vi "Ballard 429 - Build Message.vi"(0 "Channel Data []":T5[](array[typedef])=[{"Labels Settings"=[{"Name"="", "xmlName"="", "Label"=0, "transferPeriod"=0, "SDI_Enabled"=FALSE, "SDI"=0, "Word"={"Param Setting"={"Start Bit"=[], "Num Bits"=[], "Signed?"=[], "ScaleFac"=[], "ScaleOffset"=[], "Block Data Refs"=[], "Encoding"=[], "Values Array"=[], "Item Refs"=[]}}, "TransferType"=enum."ScheduledLabel", "has timestamp?"=FALSE, "Label Disable/Trigger Channel Reference"=0, "Message Handle"=0, "Initialized?"=FALSE, "Word Initial Raw Value"=0, "Label Timestamp Channel Data Reference"=0}], "channel handle"=0, "channel #"=0}] {"Labels Settings"."Label Timestamp Channel Data Reference" format="%.0x"; "Labels Settings"."Label Disable/Trigger Channel Reference" format="%.0x"; "Labels Settings"."Word"."Param Setting"."Item Refs" format="%.0x"; "Labels Settings"."Word"."Param Setting"."Num Bits" min=1 max=32; "Labels Settings"."Word"."Param Setting"."Start Bit" min=8 max=31; "Labels Settings"."Label" format="%.0o"}, 5 "Doubles []":dbl[](array[numeric]), 9 "Updated FIFO Index []":i32[](array[numeric]), 11 "Error (in)":errorcluster, 12 "Map":T4[](array[typedef]) {"Channel Data Reference" format="%.0x"}, 13 "Raw Values":T1) -> (15 "Error (out)":errorcluster)   [LabVIEW 2019, in "Ballard Arinc-429 Engine.lvlib"]
uses:
  Ballard Arinc-429 Engine.lvlib
  Shared/Controls and Global/RT HW Channel.ctl
  Shared/Controls and Global/RT Label Settings.ctl
  Shared/Controls and Global/Label.ctl
  Shared/Controls and Global/transferPeriod.ctl
  Shared/Controls and Global/RT Word Settings.ctl
  Shared/Controls and Global/RT Param Setting.ctl
  Shared/Controls and Global/Start Bit.ctl
  Shared/Controls and Global/Number of Bits.ctl
  <vilib>/NI VeriStand/Custom Device API/Block Data Reference.ctl
  <vilib>/NI VeriStand/Custom Device API/Data Reference.ctl
  <vilib>/NI VeriStand/Custom Device API/Custom Device Item Ref.ctl
  Shared/Controls and Global/TransferType.ctl
  RT Controls/RT Tx Association.ctl
  RT Controls/RT Tx Default Raw Value.ctl
  RT Controls/RT Tx Default Raw Value_Association.ctl
  Insert BCD Parameter.vi
  <instrlib>/BTI429Lib/BTI429LV.lvlib
  <vilib>/NI VeriStand/Custom Device Tools/Custom Device Utility Library/Custom Device Utility Library.lvlib
  Shared/Ballard Arinc-429 Shared.lvlib
  <vilib>/NI VeriStand/Custom Device API/Custom Device API.lvlib
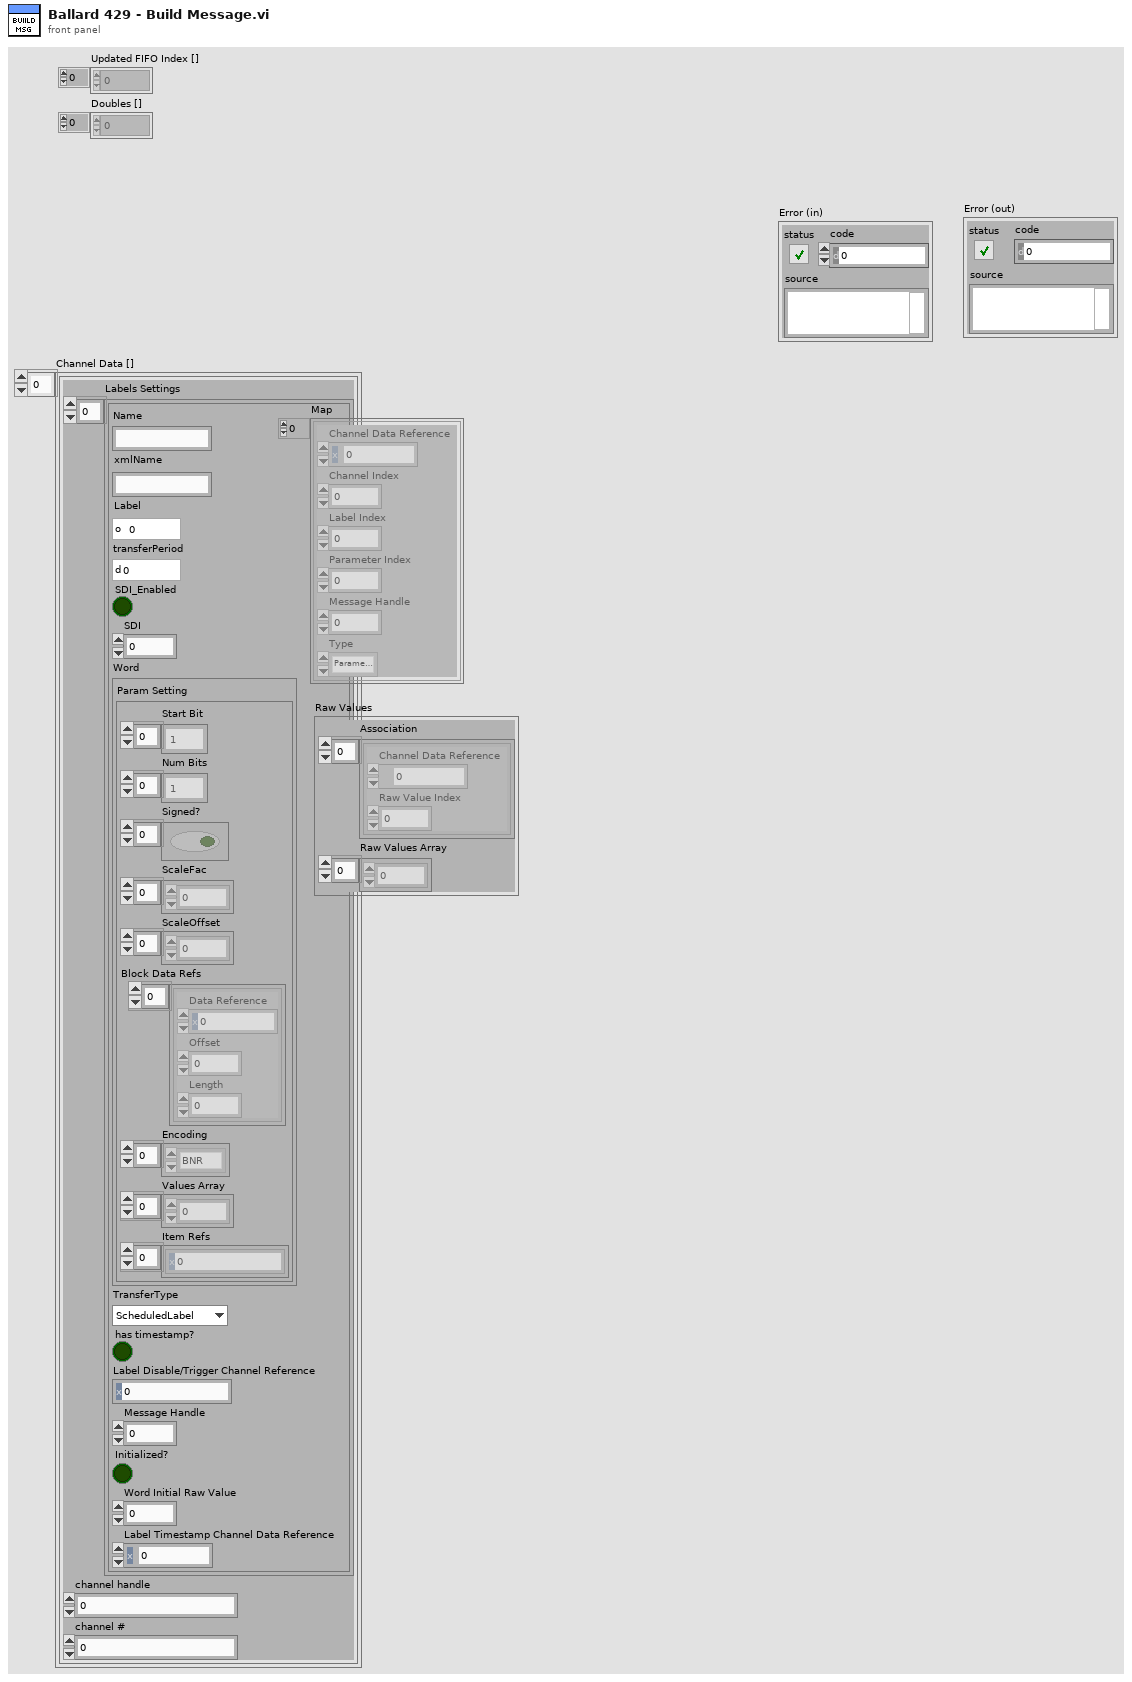
[diagram p1: front panel]
types:
  T1 = typedef "Ballard Arinc-429 Engine.lvlib/RT Tx Default Raw Value.ctl" = cluster{"Association":T2[], "Raw Values Array":u32[]}
  T2 = typedef "Ballard Arinc-429 Engine.lvlib/RT Tx Default Raw Value_Association.ctl" = cluster{"Channel Data Reference":T3, "Raw Value Index":i32}
  T3 = typedef "Custom Device API.lvlib/Data Reference.ctl" = i32
  T4 = typedef "Ballard Arinc-429 Engine.lvlib/RT Tx Association.ctl" = cluster{"Channel Data Reference":T3, "Channel Index":i32, "Label Index":i32, "Parameter Index":i32, "Message Handle":u64, "Type":enum16{"Parameter Channel", "Disable/Trigger Channel"}}
  T5 = typedef "Ballard Arinc-429 Shared.lvlib/RT HW Channel.ctl" = cluster{"Labels Settings":T6[], "channel handle":u64, "channel #":u16}
  T6 = typedef "Ballard Arinc-429 Shared.lvlib/RT Label Settings.ctl" = cluster{"Name":string, "xmlName":string, "Label":T7, "transferPeriod":T8, "SDI_Enabled":bool, "SDI":u8, "Word":T9, "TransferType":T15, "has timestamp?":bool, "Label Disable/Trigger Channel Reference":T14, "Message Handle":u64, "Initialized?":bool, "Word Initial Raw Value":u32, "Label Timestamp Channel Data Reference":T3}
  T7 = typedef "Ballard Arinc-429 Shared.lvlib/Label.ctl" = u8
  T8 = typedef "Ballard Arinc-429 Shared.lvlib/transferPeriod.ctl" = u32
  T9 = typedef "Ballard Arinc-429 Shared.lvlib/RT Word Settings.ctl" = cluster{"Param Setting":T10}
  T10 = typedef "Ballard Arinc-429 Shared.lvlib/RT Param Setting.ctl" = cluster{"Start Bit":T11[], "Num Bits":T12[], "Signed?":bool[], "ScaleFac":dbl[], "ScaleOffset":dbl[], "Block Data Refs":T13[], "Encoding":enum16{"BNR", "BCD", "Discrete"}[], "Values Array":dbl[], "Item Refs":T14[]}
  T11 = typedef "Ballard Arinc-429 Shared.lvlib/Start Bit.ctl" = i32
  T12 = typedef "Ballard Arinc-429 Shared.lvlib/Number of Bits.ctl" = i32
  T13 = typedef "Custom Device API.lvlib/Block Data Reference.ctl" = cluster{"Data Reference":T3, "Offset":u64, "Length":u64}
  T14 = typedef "Custom Device API.lvlib/Custom Device Item Ref.ctl" = u64
  T15 = typedef "Ballard Arinc-429 Shared.lvlib/TransferType.ctl" = enum16{"ScheduledLabel", "Acyclic", "Block", "Strobe"}
  T16 = enum16{"Parameter Channel", "Disable/Trigger Channel"}
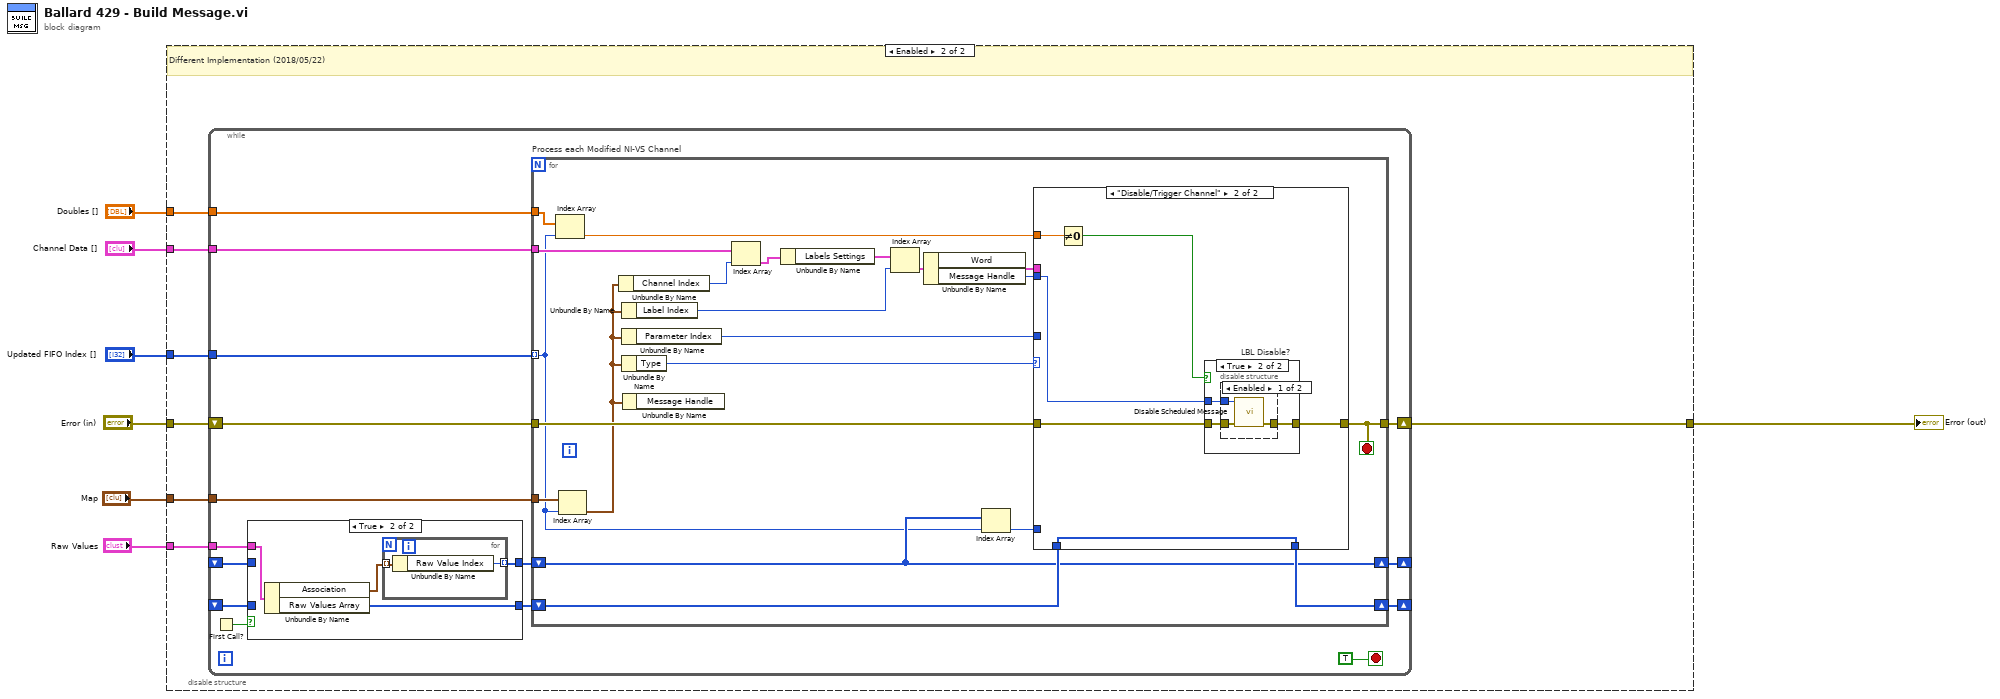
[diagram p0: block diagram]
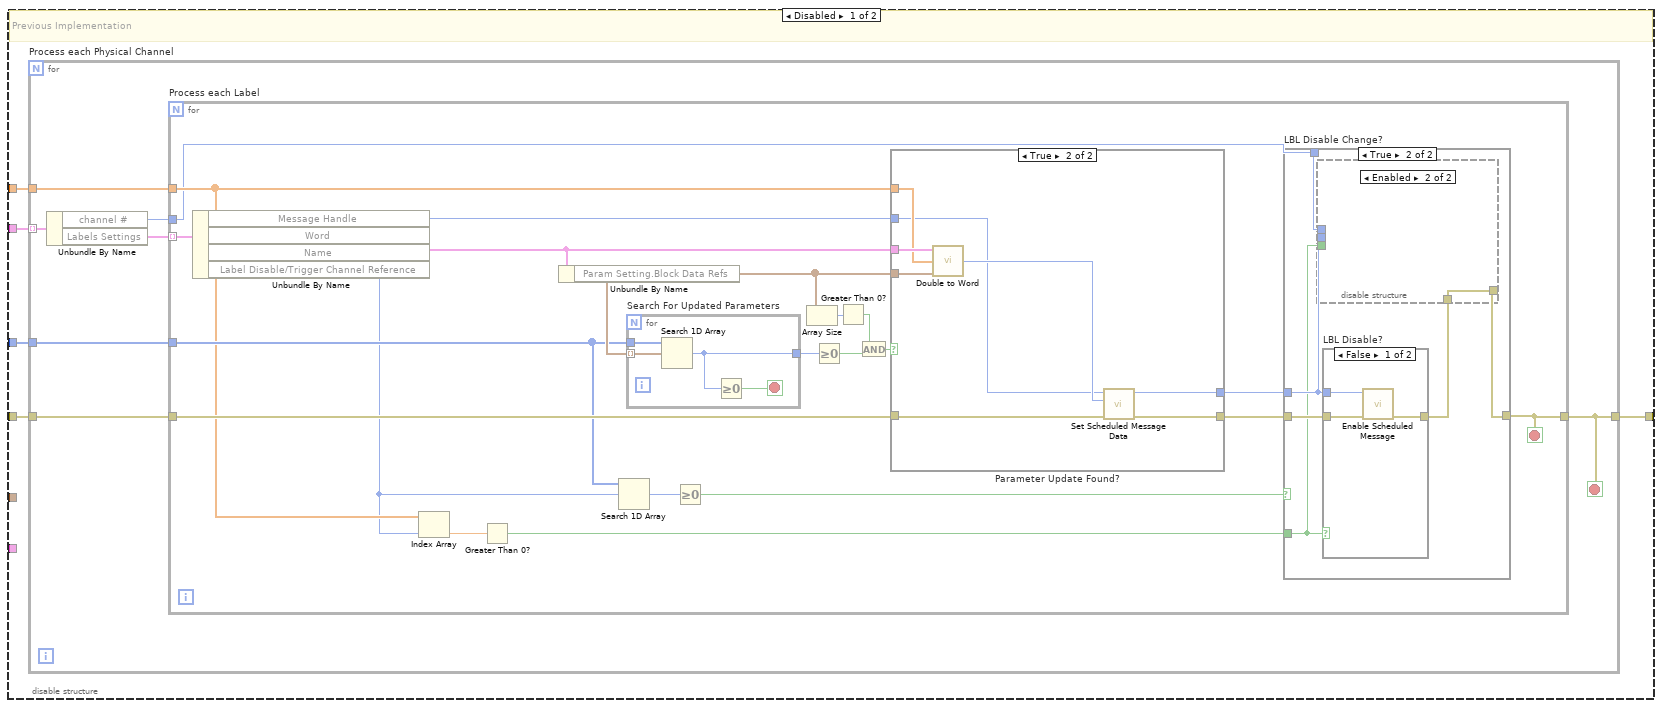
[diagram p2: hidden frame]
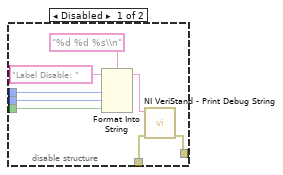
[diagram p4: hidden frame]
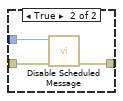
[diagram p5: hidden frame]
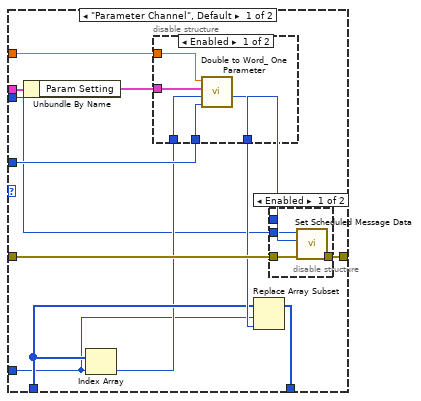
[diagram p8: hidden frame]
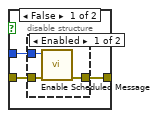
[diagram p11: hidden frame]
diagram:
  n1 = disable-structure shown="Enabled" {
    disable-tunnel: "Channel Data []" -> [w12 w83]
    disable-tunnel: "Updated FIFO Index []" -> [w11 w82]
    disable-tunnel: "Error (in)" -> [w10 w81]
    disable-tunnel: [w9 w80] -> w4
    disable-tunnel: "Doubles []" -> [w8 w79]
    disable-tunnel: "Map" -> [_ w78]
    disable-tunnel: "Raw Values" -> [_ w77]
    frame Disabled {
      # "Previous Implementation"
      n2 = for "Process each Physical Channel" {
        tunnel: w12 -> [w19] mode=indexing
        tunnel: w11 -> [w17]
        tunnel: w8 -> [w16]
        tunnel: w10 -> [w15]
        tunnel: [w14] -> w9
        stop <- w14 stop-if-true
        n3 = Unbundle By Name(w19) -> ("channel #"=w13:u16, "Labels Settings"=w18:T6[])
        n4 = for "Process each Label" {
          tunnel: w18 -> [w40] mode=indexing
          tunnel: w17 -> [w32]
          tunnel: w16 -> [w27]
          tunnel: [w29] -> w14
          tunnel: w15 -> [w38]
          tunnel: w13 -> [w21]
          stop <- w29 stop-if-true
          n5 = Unbundle By Name(w40) -> ("Message Handle"=w22:u64, "Word"=w20:T9, "Label Disable/Trigger Channel Reference"=w26:T14)  [unwired: 1 out]
          n6 = Index Array(array=w27, index=w26) -> (element=w25:dbl)
          n7 = Greater Than 0?(x=w25) -> (x > 0?=w24:bool)
          n8 = Unbundle By Name(w20) -> ("Param Setting.Block Data Refs"=w37:T13[])
          n9 = Search 1D Array(1D array=w32, element=w26) -> (index of element=w31:i32)  [unwired: 1 in]
          n10 = for "Search For Updated Parameters" {
            tunnel: w32 -> [w76]
            tunnel: w37 -> [w75] mode=indexing
            tunnel: [w74] -> w39
            stop <- w73 stop-if-true
            n11 = Search 1D Array(1D array=w76, element=w75) -> (index of element=w74:i32)  [unwired: 1 in]
            n12 = Greater Or Equal To 0?(x=w74) -> (x >= 0?=w73:bool)
          }
          n13 = Greater Or Equal To 0?(x=w31) -> (x >= 0?=w30:bool)
          n14 = Array Size(array=w37) -> (size(s)=w36:i32)
          n15 = Greater Or Equal To 0?(x=w39) -> (x >= 0?=w34:bool)
          n16 = Greater Than 0?(x=w36) -> (x > 0?=w35:bool)
          n17 = And(x=w35, y=w34) -> (x .and. y?=w33:bool)
          n18 = case "Parameter Update Found?" shown="True" w33 {
            tunnel: w27 -> [_ w68]
            tunnel: w20 -> [_ w72]
            tunnel: w38 -> [w64 w67]
            tunnel: [w64 w71] -> w28
            tunnel: w37 -> [_ w69]
            tunnel: w22 -> [w63 w66]
            tunnel: [w63 w65] -> w23
            frame False {
            }
            frame True {
              n19 = call "Double to Word.vi"("Word"=w72, "Doubles In []"=w68, "Channel FIFO Buffer Index"=w69) -> ("Word"=w70:u32)  [unwired: 12 in]
              n20 = call <instrlib>:"Set Scheduled Message Data.vi"("error in (no error)"=w67, "value"=w70, "message handle in"=w66) -> ("error out"=w71:errorcluster, "message handle out"=w65:u64)  [unwired: 7 in]
            }
          }
          n21 = case "LBL Disable Change?" shown="True" w30 {
            tunnel: [w41 w46] -> w29
            tunnel: w28 -> [w41 w47]
            tunnel: w24 -> [_ w42]
            tunnel: w23 -> [_ w43]
            tunnel: w21 -> [_ w44]
            frame False {
            }
            frame True {
              n22 = case "LBL Disable?" shown="False" w42 {
                tunnel: [w59 w62] -> w45
                tunnel: w47 -> [w58 w61]
                tunnel: w43 -> [w57 w60]
                frame False {
                  n23 = call <instrlib>:"Enable Scheduled Message.vi"("error in (no error)"=w58, "message handle in"=w57) -> ("error out"=w59:errorcluster)  [unwired: 8 in, 1 out]
                }
                frame True {
                  n24 = call <instrlib>:"Disable Scheduled Message.vi"("error in (no error)"=w61, "message handle in"=w60) -> ("error out"=w62:errorcluster)  [unwired: 8 in, 1 out]
                }
              }
              n25 = disable-structure shown="Enabled" {
                disable-tunnel: [w55 w56] -> w46
                disable-tunnel: w45 -> [w54 w56]
                disable-tunnel: w44 -> [w51 _]
                disable-tunnel: w43 -> [w50 _]
                disable-tunnel: w42 -> [w49 _]
                frame Disabled {
                  n26 = Format Into String(format string="%d %d %s\\n", initial string="Label Disable: ", w51, w50, w49) -> (resulting string=w52:string)  [unwired: 1 in, 1 out]
                  n27 = call <vilib>:"NI VeriStand - Print Debug String.vi"("error in (no error)"=w54, "Message"=w52) -> ("error out"=w55:errorcluster)  [unwired: 9 in]
                }
                frame Enabled {
                }
              }
            }
          }
        }
      }
    }
    frame Enabled {
      # "Different Implementation (2018/05/22)"
      n28 = while {
        tunnel: w83 -> [w98]
        tunnel: w82 -> [w97]
        tunnel: w79 -> [w94]
        tunnel: w78 -> [w93]
        shift-right: [w95] -> w80
        shift-left: w81 -> [w96]
        tunnel: w77 -> [w91]
        shift-right: [w89] -> _
        shift-left: _ -> [w88]
        shift-right: [w86] -> _
        shift-left: _ -> [w85]
        stop <- TRUE stop-if-true
        n29 = First Call?() -> (First Call?: T/F=w84:bool)
        n30 = case shown="True" w84 {
          tunnel: w91 -> [_ w104]
          tunnel: [w100 w103] -> w90
          tunnel: w88 -> [w100 _]
          tunnel: [w99 w101] -> w87
          tunnel: w85 -> [w99 _]
          frame False {
          }
          frame True {
            n31 = Unbundle By Name(w104) -> ("Association"=w102:T2[], "Raw Values Array"=w103:u32[])
            n32 = for {
              tunnel: w102 -> [w106] mode=indexing
              tunnel: [w105] -> w101 mode=indexing
              n33 = Unbundle By Name(w106) -> ("Raw Value Index"=w105:i32)
            }
          }
        }
        n34 = for "Process each Modified NI-VS Channel" {
          tunnel: w98 -> [w126]
          tunnel: w97 -> [w109] mode=indexing
          tunnel: w94 -> [w114]
          tunnel: w96 -> [w127]
          tunnel: [w115] -> w95
          tunnel: w93 -> [w119]
          shift-right: [w111] -> w89
          shift-left: w90 -> [w112]
          shift-right: [w110] -> w86
          shift-left: w87 -> [w110]
          stop <- w115 stop-if-true
          n35 = Index Array(array=w114, index=w109) -> (element=w113:dbl)
          n36 = Index Array(array=w119, index=w109) -> (element=w117:T4)
          n37 = Unbundle By Name(w117) -> ("Channel Index"=w125:i32)
          n38 = Unbundle By Name(w117) -> ("Label Index"=w122:i32)
          n39 = Unbundle By Name(w117) -> ("Parameter Index"=w120:i32)
          n40 = Unbundle By Name(w117) -> ("Type"=w116:T16)
          n41 = Unbundle By Name(w117) -> ()  [unwired: 1 out]
          n42 = Index Array(array=w126, index=w125) -> (element=w124:T5)
          n43 = Unbundle By Name(w124) -> ("Labels Settings"=w123:T6[])
          n44 = Index Array(array=w123, index=w122) -> (element=w121:T6)
          n45 = Unbundle By Name(w121) -> ("Word"=w118:T9, "Message Handle"=w107:u64)
          n46 = Index Array(array=w110, index=w109) -> (element=w108:i32)
          n47 = case shown="\"Disable/Trigger Channel\"" w116 {
            tunnel: w127 -> [w139 w156]
            tunnel: [w138 w155] -> w115
            tunnel: w120 -> [w131 _]
            tunnel: w118 -> [w134 _]
            tunnel: w113 -> [w133 w154]
            tunnel: w112 -> [w135 w152]
            tunnel: [w136 w152] -> w111
            tunnel: w108 -> [w129 _]
            tunnel: w107 -> [w128 w151]
            frame "Parameter Channel", Default {
              n48 = Unbundle By Name(w134) -> ("Param Setting"=w132:T10)
              n49 = Index Array(array=w135, index=w129) -> (element=w130:u32)
              n50 = disable-structure shown="Enabled" {
                disable-tunnel: [w144 w145] -> w137
                disable-tunnel: w133 -> [w143 _]
                disable-tunnel: w132 -> [w142 _]
                disable-tunnel: w131 -> [w141 _]
                disable-tunnel: w130 -> [w140 w145]
                frame Enabled {
                  n51 = call "Double to Word_ One Parameter.vi"("Parameter Index"=w141, "Word In"=w140, "Param Setting"=w142, "NI-VS Channel"=w143) -> ("Word Out"=w144:u32)  [unwired: 5 in]
                }
                frame Disabled {
                }
              }
              n52 = Replace Array Subset(array=w135, new element=w137, index=w129) -> (w136:u32[])
              n53 = disable-structure shown="Enabled" {
                disable-tunnel: w139 -> [w149 w150]
                disable-tunnel: [w148 w150] -> w138
                disable-tunnel: w137 -> [w147 _]
                disable-tunnel: w128 -> [w146 _]
                frame Enabled {
                  n54 = call <instrlib>:"Set Scheduled Message Data.vi"("error in (no error)"=w149, "value"=w147, "message handle in"=w146) -> ("error out"=w148:errorcluster)  [unwired: 7 in, 1 out]
                }
                frame Disabled {
                }
              }
            }
            frame "Disable/Trigger Channel" {
              n55 = Not Equal To 0?(x=w154) -> (x != 0?=w153:bool)
              n56 = case "LBL Disable?" shown="True" w153 {
                tunnel: [w159 w166] -> w155
                tunnel: w156 -> [w158 w165]
                tunnel: w151 -> [w157 w164]
                frame False {
                  n57 = disable-structure shown="Enabled" {
                    disable-tunnel: [w162 w163] -> w159
                    disable-tunnel: w158 -> [w161 w163]
                    disable-tunnel: w157 -> [w160 _]
                    frame Enabled {
                      n58 = call <instrlib>:"Enable Scheduled Message.vi"("error in (no error)"=w161, "message handle in"=w160) -> ("error out"=w162:errorcluster)  [unwired: 8 in, 1 out]
                    }
                    frame Disabled {
                    }
                  }
                }
                frame True {
                  n59 = disable-structure shown="Enabled" {
                    disable-tunnel: [w169 w170] -> w166
                    disable-tunnel: w165 -> [w168 w170]
                    disable-tunnel: w164 -> [w167 _]
                    frame Enabled {
                      n60 = call <instrlib>:"Disable Scheduled Message.vi"("error in (no error)"=w168, "message handle in"=w167) -> ("error out"=w169:errorcluster)  [unwired: 8 in, 1 out]
                    }
                    frame Disabled {
                    }
                  }
                }
              }
            }
          }
        }
      }
    }
  }
  "Error (out)" <- w4
